vi "LaserLineDetection_Intensity_SampledSearch.vi"(0 "Image In":T1, 5 "Region of Interest (Rectangle)":T2, 7 "Image Center (Horizontal)":i32, 9 "Samples":cluster{"Amount (odd)":i32, "Distance":i32}, 11 "error in (no error)":errorcluster) -> (4 "Image Out":T1, 6 "slope SS":dbl, 8 "intercept SS":dbl, 10 "INTENSITYarray SS":u8[](array[numeric]), 12 "appended array Imax":cluster{u8[], i32[]}[][](array[cluster]), 13 "appended array Gauss":cluster{u8[], i32[]}[][](array[cluster]), 14 "Sampled Search Accepted":bool, 15 "error out":errorcluster)   [LabVIEW 2013]
uses:
  <vilib>/vision/Image Controls.llb/IMAQ Image.ctl
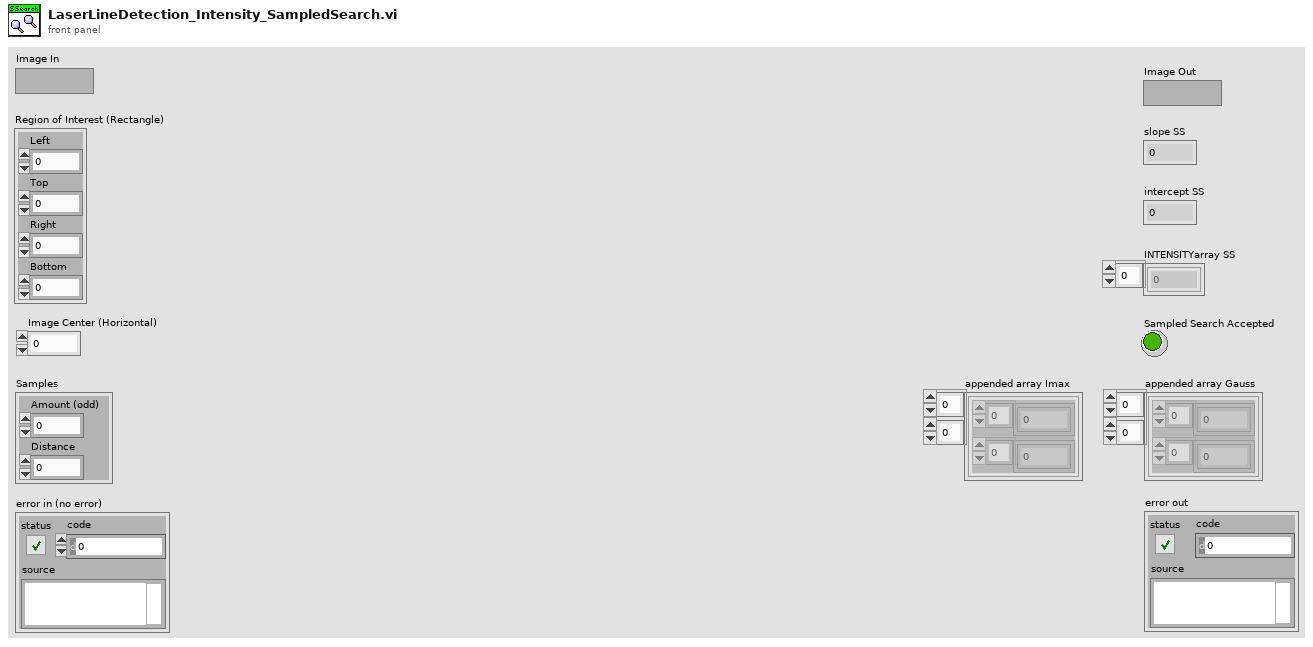
[diagram p1: front panel]
types:
  T1 = typedef "IMAQ Image.ctl" = refnum<image>
  T2 = cluster{"Left":i32, "Top":i32, "Right":i32, "Bottom":i32}
  T3 = typedef "Point Information.ctl" = cluster{"X":i32, "Y":i32, "Intensity":u8}
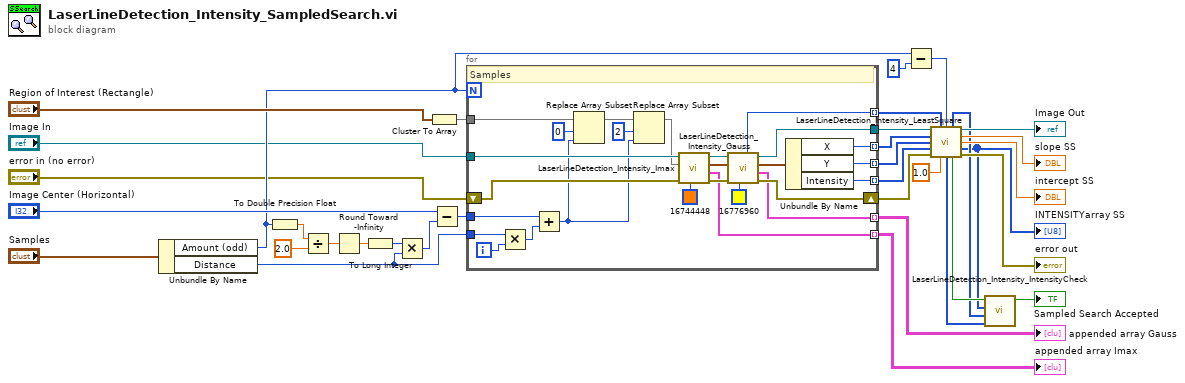
[diagram p0: block diagram]
diagram:
  n1 = Unbundle By Name("Samples") -> ("Amount (odd)"=w18:i32, "Distance"=w33:i32)
  n2 = To Double Precision Float(number=w18) -> (double precision float=w10:dbl)
  n3 = Divide(x=w10, y=2.0) -> (x/y=w12:dbl)
  n4 = Round Toward -Infinity(1:w12) -> (0:w13:dbl)
  n5 = To Long Integer(number=w13) -> (32bit integer=w9:i32)
  n6 = Multiply(x=w9, y=w33) -> (x*y=w8:i32)
  n7 = Cluster To Array(cluster="Region of Interest (Rectangle)") -> (array=w15:i32[])
  n8 = Subtract(x="Image Center (Horizontal)", y=w8) -> (x-y=w14:i32)
  n9 = for {
    N: w18 -> [_]
    tunnel: w14 -> [w61]
    tunnel: w33 -> [w59]
    tunnel: w15 -> [w57]
    tunnel: "Image In" -> [w52]
    shift-right: [w46] -> w22
    shift-left: "error in (no error)" -> [w53]
    tunnel: [w47] -> w21
    tunnel: [w43] -> w23 mode=indexing
    tunnel: [w42] -> w24 mode=indexing
    tunnel: [w41] -> w25 mode=indexing
    tunnel: [w38] -> w34 mode=indexing
    tunnel: [w37] -> w35 mode=indexing
    tunnel: [w36] -> w6 mode=indexing
    i -> [w60]
    # "Samples"
    n10 = Multiply(x=w59, y=w60) -> (x*y=w58:i32)
    n11 = Add(x=w61, y=w58) -> (x+y=w50:i32)
    n12 = Replace Array Subset(array=w57, new element=w50, index=0) -> (w54:i32[])
    n13 = Replace Array Subset(array=w54, new element=w50, index=2) -> (w51:i32[])
    n14 = call "LaserLineDetection_Intensity_Imax.vi"("Color"=u32 16744448, "error in (no error)"=w53, "Line Coordinates"=w51, "Image In"=w52) -> ("error out"=w49:errorcluster, "appended array"=w38:cluster{u8[], i32[]}[], "Point Information"=w45:T3, "Image Out"=w48:T1)  [unwired: 4 in]
    n15 = call "LaserLineDetection_Intensity_Gauss.vi"("Color"=u32 16776960, "Error In"=w49, "Point Information In"=w45, "Source In"=w48) -> ("Error Out"=w46:errorcluster, "appended array"=w37:cluster{u8[], i32[]}[], "Point Information Out"=w44:T3, "Source Out"=w47:T1, "Intensity Average"=w36:u8)  [unwired: 2 in, 1 out]
    n16 = Unbundle By Name(w44) -> ("X"=w43:i32, "Y"=w42:i32, "Intensity"=w41:u8)
  }
  "appended array Gauss" <- w35
  "appended array Imax" <- w34
  n17 = Subtract(x=w18, y=4) -> (x-y=w7:i32)
  n18 = call "LaserLineDetection_Intensity_LeastSquare.vi"("Image In"=w21, "I_AVERAGEarray In"=w6, "Loop Count"=w7, "Xarray In"=w23, "Yarray In"=w24, "INTENSITYarray In"=w25, "error in (no error)"=w22, "tolerance (residue)"=1.0) -> ("I_AVERAGEarray Out"=w3:u8[], "Image Out"=→"Image Out":T1, "slope"=→"slope SS":dbl, "intercept"=→"intercept SS":dbl, "INTENSITYarray Out"=w2:u8[], "Yarray Out"=w1:i32[], "Least Square Accepted"=w4:bool, "error out"=→"error out":errorcluster)
  "INTENSITYarray SS" <- w2
  n19 = call "LaserLineDetection_Intensity_IntensityCheck.vi"("Yarray"=w1, "I_AVERAGEarray"=w3, "INTENSITYarray"=w2, "Least Square Accepted"=w4) -> ("Sampled Search Accepted"=→"Sampled Search Accepted":bool)  [unwired: 7 in]
